vi "nominal run update set start.vi"(8 "error in (no error)":errorcluster, 10 "start_ms":dbl, 11 "staging":i32) -> (0 "error out":errorcluster, 3 "function return":i32)   [LabVIEW 2020, in "client.lvlib"]
doc: "int32_t nominal_run_update_set_start(int32_t staging, double start_ms);"
uses:
  client.lvlib
  nominalClient_64.dll
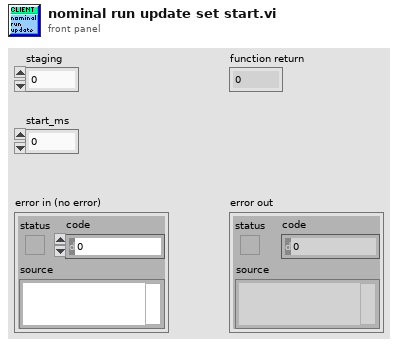
[diagram p1: front panel]
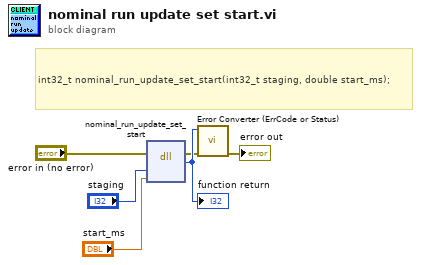
[diagram p0: block diagram]
diagram:
  # "int32_t nominal_run_update_set_start(int32_t staging, double start_ms);"
  n1 = dll-call lib="C:/code/labview-client-rs/lv_src/client/nominalClient_64.*" fn="nominal_run_update_set_start"(error in="error in (no error)", "staging"="staging", "start_ms"="start_ms") -> (error out=w2:errorcluster, w6:i32)  [unwired: 4 in, 1 out]
  "function return" <- w6
  n2 = call "Error Converter (ErrCode or Status).vi"("error in (no error)"=w2, "error code"=w6) -> ("error out"=→"error out":errorcluster)  [unwired: 9 in]
